vi "DeviceDataToTable.vi"(5 "Table History ref":refnum<vi>, 6 "Defer Updates? (T)":bool=TRUE, 7 "Table Ref In":refnum<vi>, 8 "error in (no error)":errorcluster, 9 "Col Length":i32, 10 "Index Start":i32, 11 "Device object":refnum<class "Device.lvclass">) -> (0 "error out":errorcluster)   [LabVIEW 2013]
doc: "Acting directly on the referenced table, this subVI pushes a particular devices data to the table. Checks include (i) Data rows match table rows, (ii) # data columns matches deivice Cols; each of these will throw a dialog warning the user."
uses:
  Device/Device.lvclass
  TypeDefs/TableHistory.ctl
  TypeDefs/TableArray.ctl
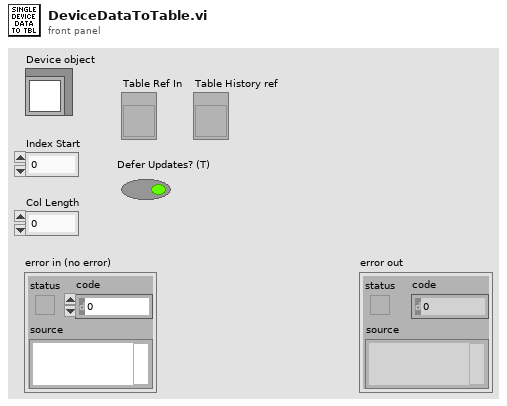
[diagram p1: front panel]
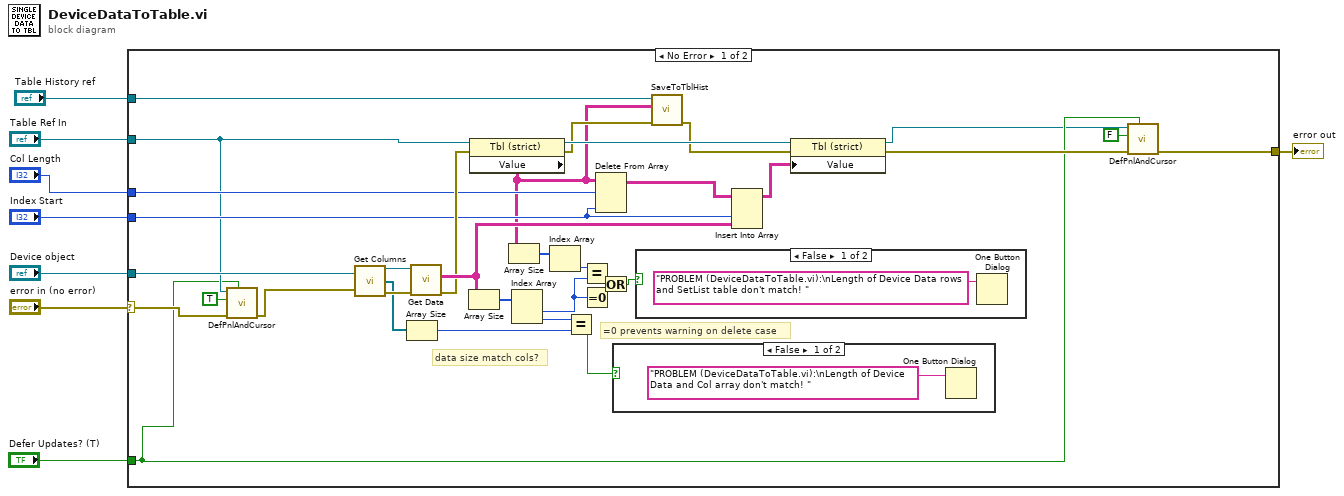
[diagram p0: block diagram]
diagram:
  n1 = case shown="No Error" "error in (no error)" {
    selector: "error in (no error)" -> [w17 w45]
    tunnel: "Table Ref In" -> [w15 _]
    tunnel: "Col Length" -> [w36 _]
    tunnel: "Index Start" -> [w35 _]
    tunnel: [w12 w45] -> w5
    tunnel: "Device object" -> [w34 _]
    tunnel: "Defer Updates? (T)" -> [w11 _]
    tunnel: "Table History ref" -> [w19 _]
    frame No Error {
      # "=0 prevents warning on delete case"
      # "data size match cols?"
      n2 = call "DefPnlAndCursor.vi"("AllowDefPan? (T)"=w11, "error in (no error)"=w17, "DeferPanUpdts?"=TRUE, "Tbl Ctrl Refnum"=w15) -> ("error out"=w16:errorcluster)  [unwired: 7 in]
      n3 = call-dynamic "Get Columns.vi"("Device in"=w34, "error in (no error)"=w16) -> ("Device out"=w33:refnum<class "Device.lvclass">, "Columns"=w31:refnum<class "Column.lvclass">[], "error out"=w32:errorcluster)
      n4 = Array Size(array=w31) -> (size(s)=w28:i32)
      n5 = call-dynamic "Get Data.vi"("error in (no error)"=w32, "Device in"=w33) -> ("error out"=w37:errorcluster, "Table Indicator"=w39:string[][])  [unwired: 6 in, 1 out]
      n6 = Array Size(array=w39) -> (size(s)=w38:i32[])
      n7 = property class="Tbl (strict)"(reference=w15, error in=w37) -> (reference out=w41:refnum<vi>, error out=w21:errorcluster, "Value"=w18:string[][])
      n8 = Array Size(array=w18) -> (size(s)=w30:i32[])
      n9 = Index Array(array=w38) -> (element #1=w25:i32, element #2=w27:i32)  [unwired: 2 in]
      n10 = Index Array(array=w30) -> (element=w29:i32)  [unwired: 1 in]
      n11 = Equal?(x=w27, y=w28) -> (x = y?=w26:bool)
      n12 = Equal?(x=w29, y=w25) -> (x = y?=w23:bool)
      n13 = Equal To 0?(x=w25) -> (x = 0?=w22:bool)
      n14 = Delete From Array "Delete From Array"(array=w18, length=w36, index (col)=w35) -> (array with subset deleted=w42:string[][])  [unwired: 1 in, 1 out]
      n15 = Or(x=w23, y=w22) -> (x .or. y?=w24:bool)
      n16 = case shown="False" w26 {
        frame False {
          n17 = One Button Dialog(message="PROBLEM (DeviceDataToTable.vi):\nLength of Device Data and Col array don't match! ") -> ()  [unwired: 1 in, 1 out]
        }
        frame True {
        }
      }
      n18 = case shown="False" w24 {
        frame False {
          n19 = One Button Dialog(message="PROBLEM (DeviceDataToTable.vi):\nLength of Device Data rows and SetList table don't match! ") -> ()  [unwired: 1 in, 1 out]
        }
        frame True {
        }
      }
      n20 = call "SaveToTblHist.vi"("error in (no error)"=w21, "OldTable (reset)"=w18, "Table History ref"=w19) -> ("error out"=w20:errorcluster)  [unwired: 8 in]
      n21 = Insert Into Array "Insert Into Array"(array=w42, index (col)=w35, new element=w39) -> (w40:string[][])  [unwired: 1 in]
      n22 = property class="Tbl (strict)"(reference=w41, error in=w20, "Value"=w40) -> (reference out=w10:refnum<vi>, error out=w13:errorcluster)
      n23 = call "DefPnlAndCursor.vi"("AllowDefPan? (T)"=w11, "error in (no error)"=w13, "DeferPanUpdts?"=FALSE, "Tbl Ctrl Refnum"=w10) -> ("error out"=w12:errorcluster)  [unwired: 7 in]
    }
    frame Error {
    }
  }
  "error out" <- w5
